vi "do_immediately.vi"() -> ()   [LabVIEW 2020]
panel:
  in  "停止":bool
  in  "Dout":bool[](array[boolean])
  out "error out":errorcluster caption="错误输出"
  in  "DevIndex":i32
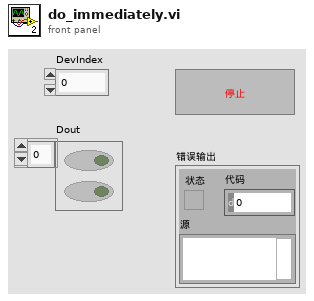
[diagram p1: front panel]
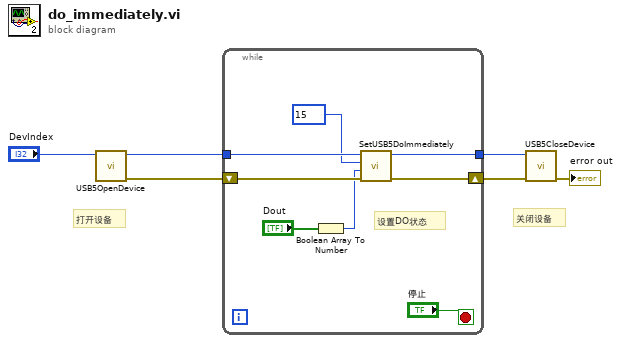
[diagram p0: block diagram]
diagram:
  # "关闭设备"
  # "打开设备"
  n1 = call "USB5OpenDevice.vi"("DevIndex"="DevIndex") -> ("error out"=w1:errorcluster, "DevIndex Out"=w2:i32)  [unwired: 9 in]
  n2 = while {
    shift-right: [w11] -> w3
    shift-left: w1 -> [w13]
    tunnel: w2 -> [w14]
    tunnel: [w12] -> w4
    stop <- "停止" stop-if-true
    # "设置DO状态"
    n3 = Boolean Array To Number(Boolean array="Dout") -> (number=w9:u32)
    n4 = call "SetUSB5DoImmediately.vi"("错误输入（无错误）"=w13, "Value"=w9, "Chan"=u32 15, "DevIndex"=w14) -> ("错误输出"=w11:errorcluster, "DevIndex Out"=w12:i32)  [unwired: 6 in]
  }
  n5 = call "USB5CloseDevice.vi"("错误输入（无错误）"=w3, "DevIndex"=w4) -> ("error out"=→"error out":errorcluster)  [unwired: 8 in, 1 out]
